vi "ApplyLayoutToObject.vi"(5 "scaling settings":T1={"scaling factor"={"horizontal"=1.0, "vertical"=1.0}, "scale text"=FALSE} {"scaling factor"."vertical" min=0.0; "scaling factor"."horizontal" min=0.0}, 7 "properties to ignore":variant, 8 "error in (no error)":errorcluster, 10 "GObj Refnum":refnum<vi>, 11 "Subpanel Control Layout in":refnum<class "Subpanel Control Layout.lvclass">) -> (0 "error out":errorcluster, 3 "Subpanel Control Layout out":refnum<class "Subpanel Control Layout.lvclass">)   [LabVIEW 2012, in "NI_SE_Front Panel Layout.lvlib" / "Subpanel Control Layout.lvclass"]
doc: "Apply layout information to the GObj Refnum."
uses:
  Subpanel Control Layout.lvclass
  Scaling Factor_Options.ctl
  XY Scaling Factor.ctl
  Control Layout/Control Layout.lvclass
  NI_SE_Front Panel Layout.lvlib
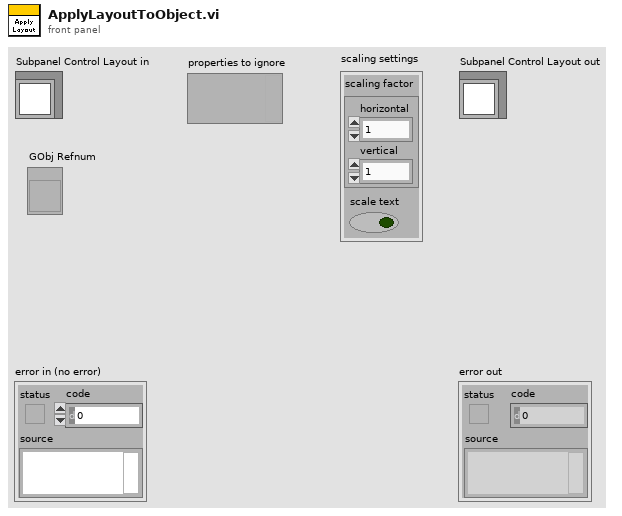
[diagram p1: front panel]
types:
  T1 = typedef "NI_SE_Front Panel Layout.lvlib/Scaling Factor_Options.ctl" = cluster{"scaling factor":T2, "scale text":bool}
  T2 = typedef "NI_SE_Front Panel Layout.lvlib/XY Scaling Factor.ctl" = cluster{"horizontal":dbl, "vertical":dbl}
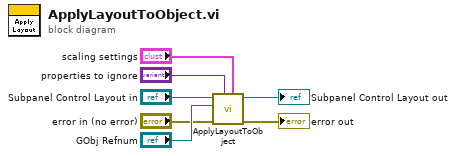
[diagram p0: block diagram]
diagram:
  n1 = call-parent "ApplyLayoutToObject.vi"("scaling settings"="scaling settings", "properties to ignore"="properties to ignore", "error in (no error)"="error in (no error)", "GObj Refnum"="GObj Refnum", "Control Layout in"="Subpanel Control Layout in") -> ("error out"=→"error out":errorcluster, "Control Layout out"=→"Subpanel Control Layout out":refnum<class "Subpanel Control Layout.lvclass">)  [unwired: 5 in]
